vi "Read error.vi"(8 "error in (no error)":errorcluster, 11 "Msg_Error.lvclass in":refnum<class "Msg_Error.lvclass">) -> (0 "error out":errorcluster, 2 "error":errorcluster, 3 "Msg_Error.lvclass out":refnum<class "Msg_Error.lvclass">)   [LabVIEW 2012, in "Msg_Error.lvlib" / "Msg_Error.lvclass"]
uses:
  Msg_Error.lvclass
  Msg_Error.lvclass/Msg_Error.ctl
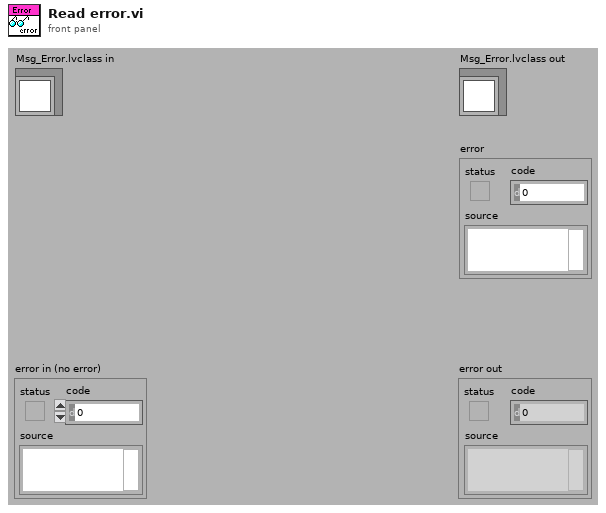
[diagram p1: front panel]
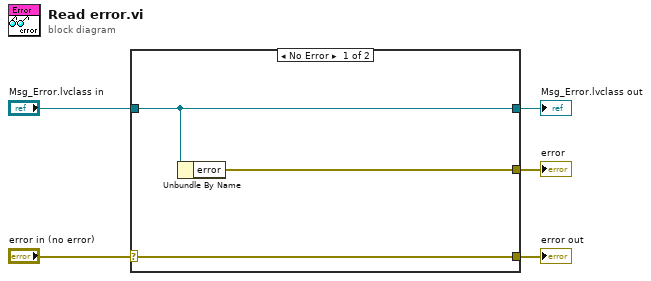
[diagram p0: block diagram]
diagram:
  n1 = case shown="No Error" "error in (no error)" {
    selector: "error in (no error)" -> [w8 w9]
    tunnel: [w8 w9] -> w4
    tunnel: [w7 w10] -> w2
    tunnel: "Msg_Error.lvclass in" -> [w7 w10]
    tunnel: [w6 _] -> w1
    frame No Error {
      n2 = Unbundle By Name(w7) -> ("error"=w6:errorcluster)
    }
    frame Error {
    }
  }
  "error out" <- w4
  "Msg_Error.lvclass out" <- w2
  "error" <- w1
